vi "Method_Const.vi"(4 "Value":i8, 5 "Input A":T1) -> (1 "Result":T1)   [LabVIEW 2021, in "Multiply_I8.lvclass"]
uses:
  Multiply_I8.lvclass
  Abs_Type.ctl
  Abs_Types/I8 Integer/Abs_I8 Integer.lvclass
  C:/Program Files (x86)/National Instruments/LabVIEW 2021/vi.lib/TSA/Abstract Data Classes/Abs_Types/Numeric/Abs_Numeric.lvclass
  C:/TSA/LV_Abstract/Source/Functions/Support/Function/Two Terminal/I8/AbsFunc_Two Term_I8.lvclass
  C:/Program Files (x86)/National Instruments/LabVIEW 2021/vi.lib/TSA/Abstract Data Classes/Abs_Types/I8 Integer/Abs_I8 Integer.lvclass
  Support/Function/Two Terminal/I8/AbsFunc_Two Term_I8.lvclass/AbsFunc_Two Term_I8.ctl
  Support/Function/Two Terminal/I8/Properties/Write Numeric A.vi
  Support/Function/Two Terminal/I8/Properties/Write Numeric B.vi
  Constants/Support/I8/Const_I8.lvclass
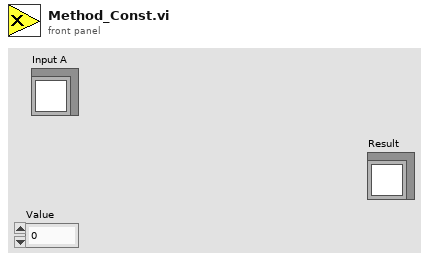
[diagram p1: front panel]
types:
  T1 = typedef "Multiply_I8.lvclass/Abs_Type.ctl" = refnum<class "Abs_I8 Integer.lvclass">
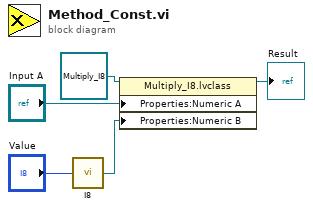
[diagram p0: block diagram]
diagram:
  n1 = call "I8.vi"("Value"="Value") -> ("Constant"=w2:refnum<class "Abs_I8 Integer.lvclass">)  [unwired: 4 in]
  n2 = property class="Multiply_I8.lvclass"(reference=refnum<class "Multiply_I8.lvclass"> refnum ("Functions.lvlib:Numeric.lvlib:Multiply.lvclass"), "Properties:Numeric A"="Input A", "Properties:Numeric B"=w2) -> (reference out=→"Result":refnum<class "Multiply_I8.lvclass">)  [unwired: 1 in, 1 out]
